vi "volume_coercer.vi"(0 "InVolume":dbl) -> (1 "OutVolume":dbl, 2 "Coerced?":bool)   [LabVIEW 2010]
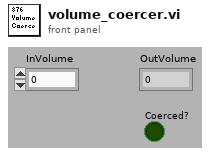
[diagram p1: front panel]
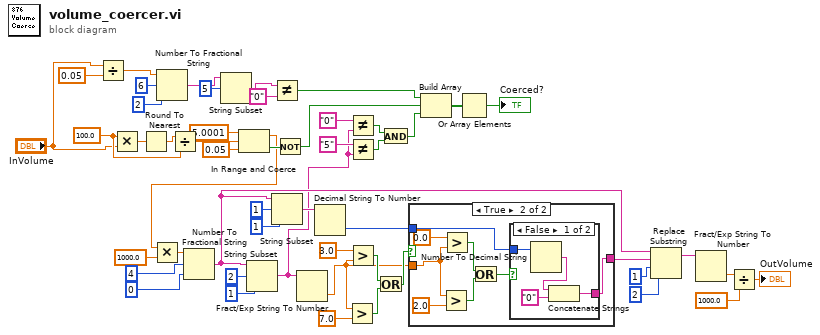
[diagram p0: block diagram]
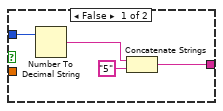
[diagram p2: hidden frame]
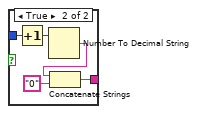
[diagram p3: hidden frame]
diagram:
  w16 = 100.0 ("x")
  n1 = Divide(x="InVolume", y=0.05) -> (x/y=w12:dbl)
  n2 = Multiply(x=w16, y="InVolume") -> (x*y=w18:dbl)
  n3 = Round To Nearest(number=w18) -> (nearest integer value=w17:dbl)
  n4 = Number To Fractional String(number=w12, width (-)=i16 6, precision (6)=i16 2) -> (F-format string=w9:string)  [unwired: 1 in]
  n5 = Divide(x=w17, y=w16) -> (x/y=w15:dbl)
  n6 = String Subset(string=w9, offset (0)=5) -> (substring=w6:string)  [unwired: 1 in]
  n7 = In Range and Coerce(upper limit=5.0001, x=w15, lower limit=0.05) -> (coerced(x)=w20:dbl, In Range?=w21:bool)
  n8 = Multiply(x=w20, y=1000.0) -> (x*y=w50:dbl)
  n9 = Number To Fractional String(number=w50, width (-)=i16 4, precision (6)=i16 0) -> (F-format string=w35:string)  [unwired: 1 in]
  n10 = String Subset(string=w35, offset (0)=2, length (rest)=1 ("length (rest)")) -> (substring=w25:string)
  n11 = Not Equal?(x=w6, y="0") -> (x != y?=w4:bool)
  n12 = String Subset(string=w35, offset (0)=1, length (rest)=1 ("length (rest)")) -> (substring=w37:string)
  n13 = Not(x=w21) -> (.not. x?=w3:bool)
  n14 = Fract/Exp String To Number(string=w25) -> (number=w40:dbl)  [unwired: 3 in, 1 out]
  n15 = Decimal String To Number(string=w37) -> (number=w36:i32)  [unwired: 2 in, 1 out]
  n16 = Greater?(x=w40, y=7.0) -> (0:w45:bool)
  n17 = Not Equal?(x="0", y=w25) -> (x != y?=w24:bool)
  n18 = Not Equal?(x="5", y=w25) -> (x != y?=w23:bool)
  n19 = Greater?(x=3.0, y=w40) -> (0:w44:bool)
  n20 = Or(x=w44, y=w45) -> (x .or. y?=w41:bool)
  n21 = And(x=w24, y=w23) -> (x .and. y?=w2:bool)
  n22 = case shown="True" w41 {
    tunnel: [w52 w63] -> w32
    tunnel: w40 -> [_ w58]
    tunnel: w36 -> [w55 w56]
    frame False {
      n23 = Number To Decimal String(number=w55) -> (decimal integer string=w53:string)  [unwired: 1 in]
      n24 = Concatenate Strings(w53, "5") -> (w52:string)
    }
    frame True {
      n25 = Greater?(x=w58, y=2.0) -> (0:w59:bool)
      n26 = Greater?(x=0.0, y=w58) -> (0:w60:bool)
      n27 = Or(x=w60, y=w59) -> (x .or. y?=w57:bool)
      n28 = case shown="False" w57 {
        tunnel: [w64 w70] -> w63
        tunnel: w56 -> [w67 w72]
        frame False {
          n29 = Number To Decimal String(number=w67) -> (decimal integer string=w65:string)  [unwired: 1 in]
          n30 = Concatenate Strings(w65, "0") -> (w64:string)
        }
        frame True {
          n31 = Increment(x=w72) -> (x+1=w71:i32)
          n32 = Number To Decimal String(number=w71) -> (decimal integer string=w69:string)  [unwired: 1 in]
          n33 = Concatenate Strings(w69, "0") -> (w70:string)
        }
      }
    }
  }
  n34 = Build Array(w4, w3, w2) -> (w1:bool[])
  n35 = Or Array Elements(Boolean array=w1) -> (logical OR=→"Coerced?":bool)
  n36 = Replace Substring(2:2 ("length (len. of substring)"), 3:1 ("offset (0)"), 4:w32, 5:w35) -> (1:w31:string)  [unwired: 1 out]
  n37 = Fract/Exp String To Number(string=w31) -> (number=w30:dbl)  [unwired: 3 in, 1 out]
  n38 = Divide(x=w30, y=1000.0) -> (x/y=→"OutVolume":dbl)
